vi "IncrementBlueSerializableVersionPathWrapper.vi"(7 "apprefnum":u32, 8 "error in (no error)":errorcluster, 9 "Version Bump 2":T1, 10 "Version Bump 1":T1, 11 "LVClass name":string) -> (0 "error out":errorcluster, 3 "BlueSerializableVersion":u16)   [LabVIEW 2019, in "IncrementMutationHistory.lvlib"]
uses:
  IncrementMutationHistory.lvlib
  <vilib>/Utility/EditLVLibs/LibVersion.ctl
  VILIB_NONUI/VILIB_NONUI.lvlib
  <vilib>/Utility/EditLVLibs/Edit LVLibs.lvlib
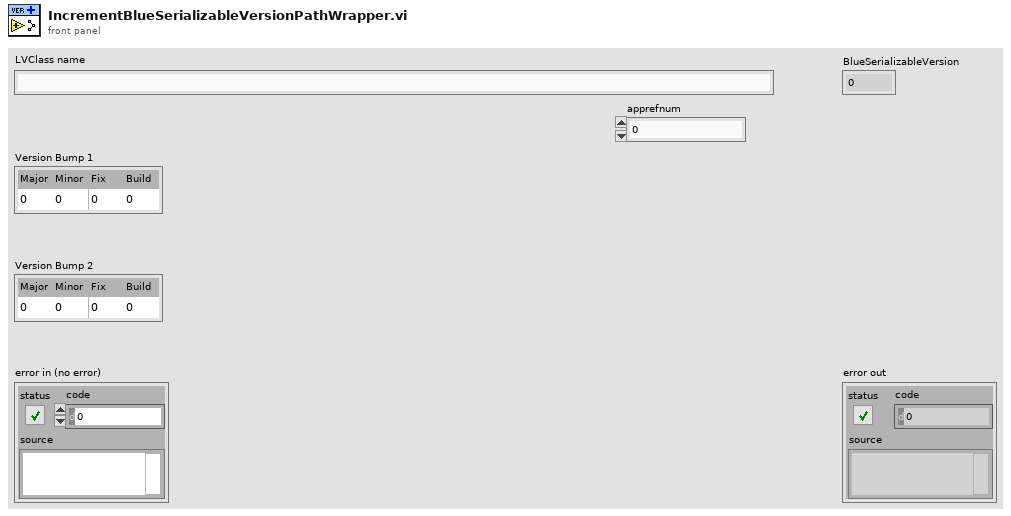
[diagram p1: front panel]
types:
  T1 = typedef "Edit LVLibs.lvlib/LibVersion.ctl" = cluster{"Major":u16, "Minor":u16, "Fix":u16, "Build":u16}
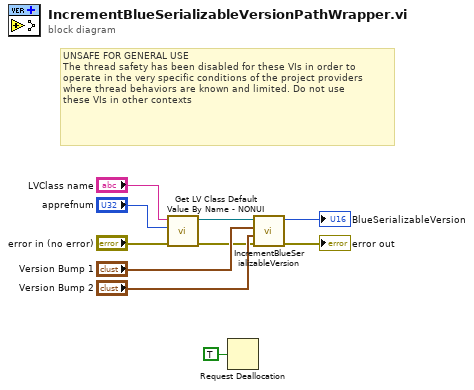
[diagram p0: block diagram]
diagram:
  # "UNSAFE FOR GENERAL USE\nThe thread safety has been disabled for these VIs in order to\noperate in the very specific conditions of the project providers\nwhere thread behaviors are known and limited. Do not use\nthese VIs in other contexts"
  n1 = call "Get LV Class Default Value By Name - NONUI.vi"("error in (no error)"="error in (no error)", "apprefnum"="apprefnum", "class name"="LVClass name") -> ("error out"=w3:errorcluster, "object"=w2:refnum<class>)  [unwired: 7 in]
  n2 = Request Deallocation(TRUE ("flag")) -> ()
  n3 = call "IncrementBlueSerializableVersion.vi"("error in (no error)"=w3, "Version Bump 2"="Version Bump 2", "Version Bump 1"="Version Bump 1", "LabVIEW Object"=w2) -> ("error out"=→"error out":errorcluster, "New BlueSerializableVersion"=→"BlueSerializableVersion":u16)  [unwired: 6 in]
